vi "SetPositionUmRealFullBit.vi"(8 "error in (no error)":errorcluster, 10 "relative Z":dbl, 11 "Stage_MadCityLab in":refnum<class "Stage_MadCityLab.lvclass">) -> (0 "error out":errorcluster, 3 "Stage_MadCityLab out":refnum<class "Stage_MadCityLab.lvclass">)   [LabVIEW 2020, in "Stage_MadCityLab.lvlib" / "Stage_MadCityLab.lvclass"]
uses:
  Stage_MadCityLab.lvclass
  Stage_MadCityLab.lvclass/Stage_MadCityLab.ctl
  Dependency/Madlib.dll
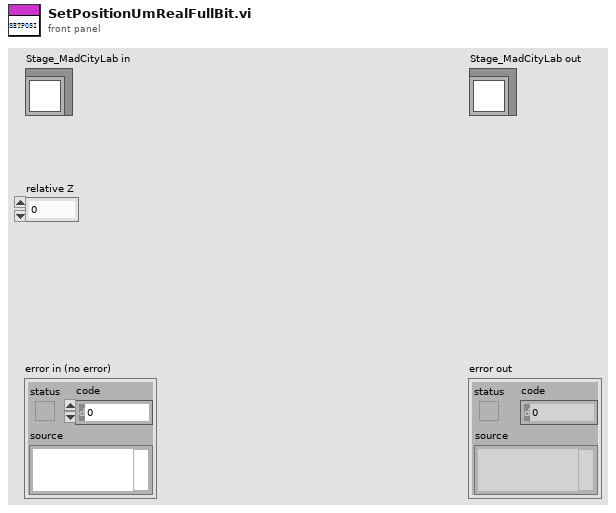
[diagram p1: front panel]
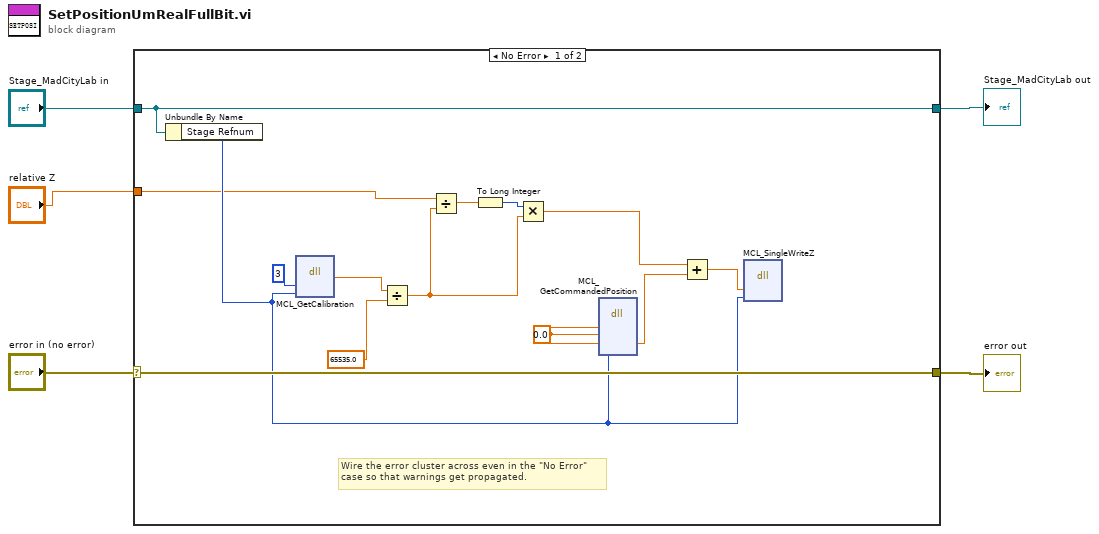
[diagram p0: block diagram]
diagram:
  n1 = case shown="No Error" "error in (no error)" {
    selector: "error in (no error)" -> [w19 w21]
    tunnel: [w19 w21] -> w4
    tunnel: [w18 w20] -> w2
    tunnel: "Stage_MadCityLab in" -> [w18 w20]
    tunnel: "relative Z" -> [w6 _]
    frame No Error {
      w10 = 0.0 ("commandX")
      # "Wire the error cluster across even in the \"No Error\"\ncase so that warnings get propagated."
      n2 = Unbundle By Name(w18) -> ("Stage Refnum"=w7:i32)
      n3 = dll-call lib="D:/Daguan/Development/MMicroscopyAF/Model/Hardware Layer/Real Hardware/Stage_MadCityLab/Stage_MadCityLab/Dependency/Madlib.dll" fn="MCL_GetCalibration"("axis"=u32 3, "handle"=w7) -> ("size"=w11:dbl)  [unwired: 5 in, 2 out]
      n4 = Divide(x=w11, y=65535.0) -> (x/y=w14:dbl)
      n5 = Divide(x=w6, y=w14) -> (x/y=w12:dbl)
      n6 = To Long Integer(number=w12) -> (32bit integer=w13:i32)
      n7 = Multiply(x=w13, y=w14) -> (x*y=w16:dbl)
      n8 = dll-call lib="D:/Daguan/Development/MMicroscopyAF/Model/Hardware Layer/Real Hardware/Stage_MadCityLab/Stage_MadCityLab/Dependency/Madlib.dll" fn="MCL_GetCommandedPosition" label="MCL_SingleReadN"("commandX"=w10, "commandY"=w10, "commandZ"=w10, "handle"=w7) -> ("commandZ"=w17:dbl)  [unwired: 5 in, 4 out]
      n9 = Add(x=w16, y=w17) -> (x+y=w15:dbl)
      n10 = dll-call lib="D:/Daguan/Development/MMicroscopyAF/Model/Hardware Layer/Real Hardware/Stage_MadCityLab/Stage_MadCityLab/Dependency/Madlib.dll" fn="MCL_SingleWriteZ"("position"=w15, "handle"=w7) -> ()  [unwired: 3 in, 5 out]
    }
    frame Error {
    }
  }
  "error out" <- w4
  "Stage_MadCityLab out" <- w2
